vi "Facade.vi"(0 "Data In":T7={"Y"={"Numeric"=25.0, "Numeric"=0.0, "Numeric"=0.0}, "end_timer"=TRUE} {"Y" scale=0.0..500.0 scale format="%#_5g"}, 2 "Display State In":T3={"SP_Source"={"connect"=FALSE, "SP_Source"=enum."initialize", "SP_Set"=0.0, "SP"=0.0}, "Write"=FALSE, "button state"=enum."init", "reset_timer"=FALSE, "load_timer"=FALSE, "end_timer"=TRUE, "Time"=0, "scale maximum"=100.0}, 3 "Container State":T6) -> (6 "Data Out":T7={"Y"={"Numeric"=25.0, "Numeric"=0.0, "Numeric"=0.0}, "end_timer"=TRUE} {"Y" scale=0.0..500.0 scale format="%#_5g"}, 7 "Display State Out":T3={"SP_Source"={"connect"=FALSE, "SP_Source"=enum."initialize", "SP_Set"=0.0, "SP"=0.0}, "Write"=FALSE, "button state"=enum."init", "reset_timer"=FALSE, "load_timer"=FALSE, "end_timer"=TRUE, "Time"=0, "scale maximum"=100.0}, 8 "Action":T2)   [LabVIEW 2019, in "Y.xctl"]
uses:
  Y.xctl
  Data.ctl
  <vilib>/_xctls/Container State.ctl
  State.ctl
  Heating/ctl/Y_source.ctl
  Y_controlState.ctl
  <vilib>/_xctls/Action.ctl
  <vilib>/_xctls/XControlSupport.lvlib
  Timer Delay/Timers.lvlib
  Heating/Heating.lvlib
panel:
  in  "setpoint":T1(slide) caption="oC" scale=0.0..500.0 scale format="%#_5g"
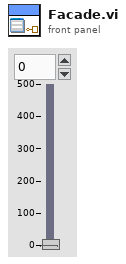
[diagram p1: front panel]
types:
  T1 = cluster{"Numeric":dbl, "Numeric":dbl, "Numeric":dbl}
  T2 = typedef "XControlSupport.lvlib/Action.ctl" = cluster{"Data Changed?":bool, "State Changed?":bool, "Action Name":string}
  T3 = typedef "Y.xctl/State.ctl" = cluster{"SP_Source":cluster{"connect":bool, "SP_Source":T4, "SP_Set":dbl, "SP":dbl}, "Write":bool, "button state":T5, "reset_timer":bool, "load_timer":bool, "end_timer":bool, "Time":u32, "scale maximum":dbl}
  T4 = typedef "Heating.lvlib/Y_source.ctl" = enum8{"initialize", "local disabled", "local hand", "hand", "auto", "dist"}
  T5 = typedef "Y.xctl/Y_controlState.ctl" = enum16{"init", "not connect", "local disabled", "local hand", "hand", "value change", "auto", "dist"}
  T6 = typedef "XControlSupport.lvlib/Container State.ctl" = cluster{"Indicator?":bool, "Run Mode?":bool, " Refnum":refnum<vi>}
  T7 = typedef "Y.xctl/Data.ctl" = cluster{"Y":cluster{"Numeric":dbl, "Numeric":dbl, "Numeric":dbl}, "end_timer":bool}
  T8 = enum8{"Enabled", "Disabled", "Disabled and Grayed Out"}
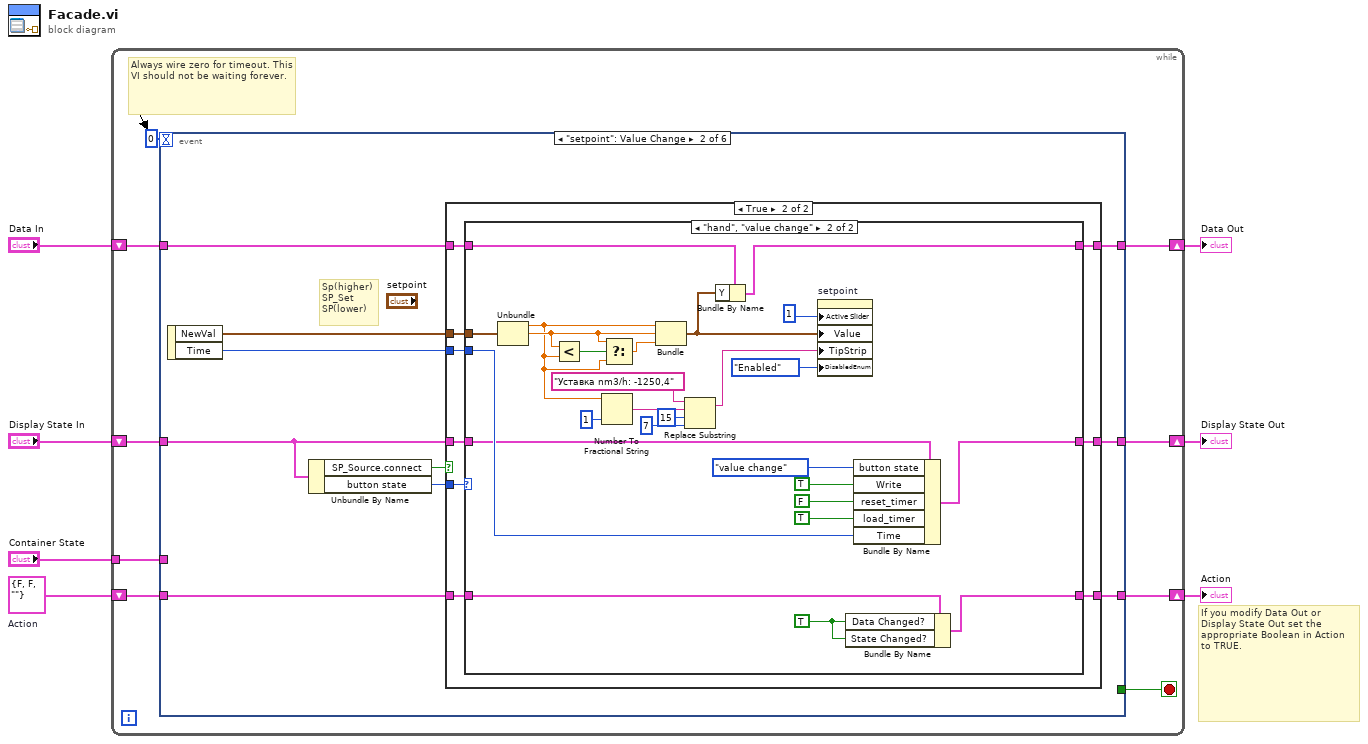
[diagram p0: block diagram]
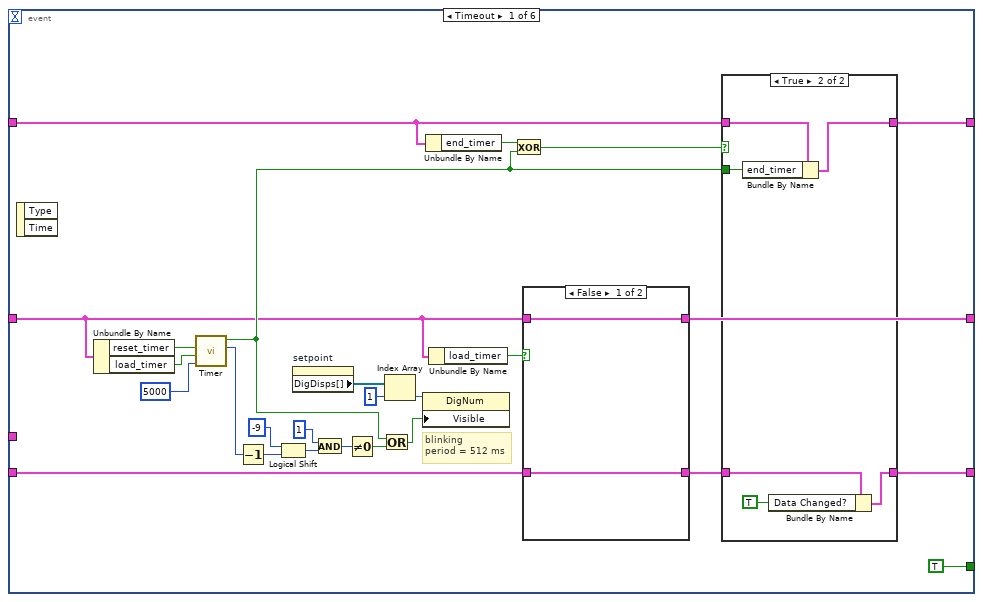
[diagram p2: hidden frame]
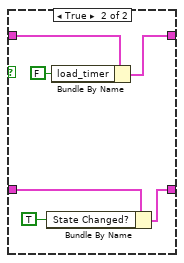
[diagram p4: hidden frame]
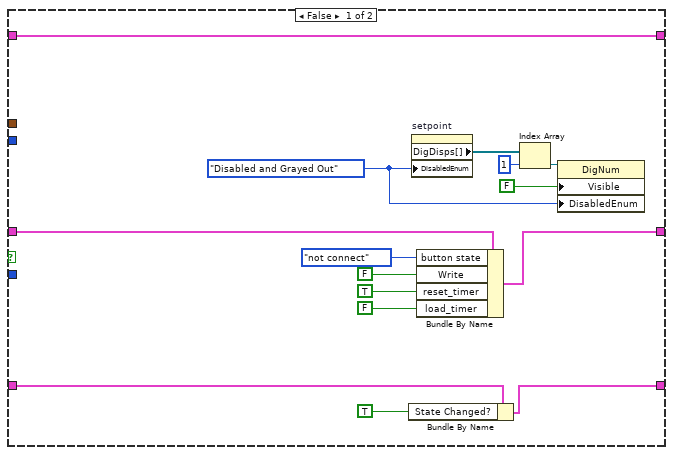
[diagram p5: hidden frame]
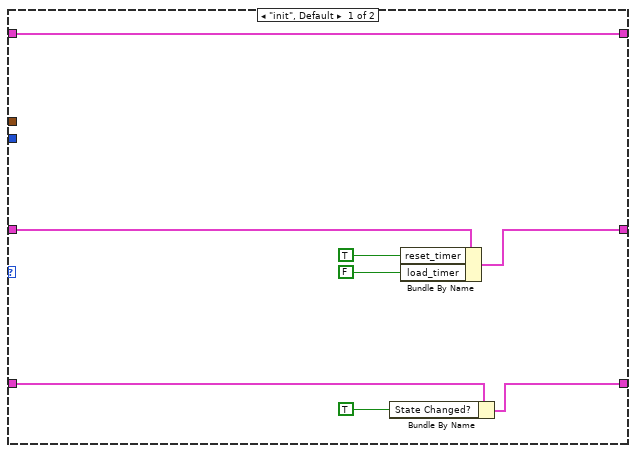
[diagram p6: hidden frame]
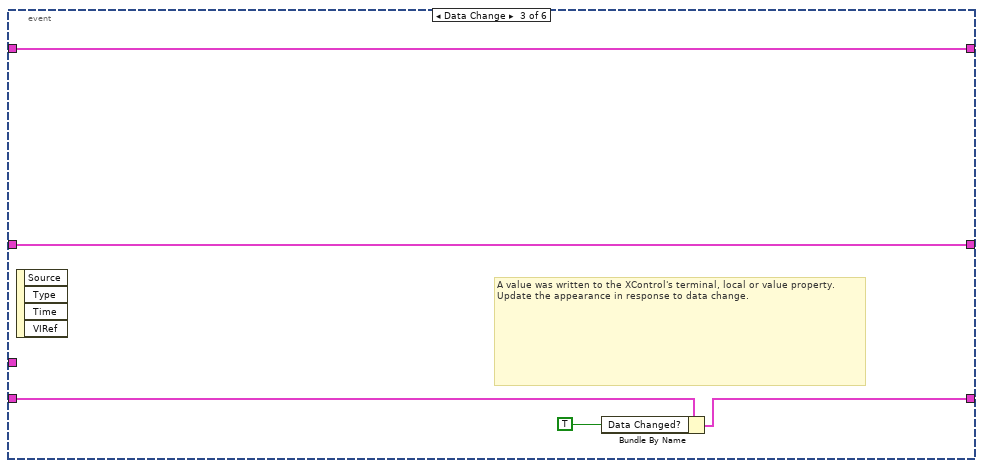
[diagram p7: hidden frame]
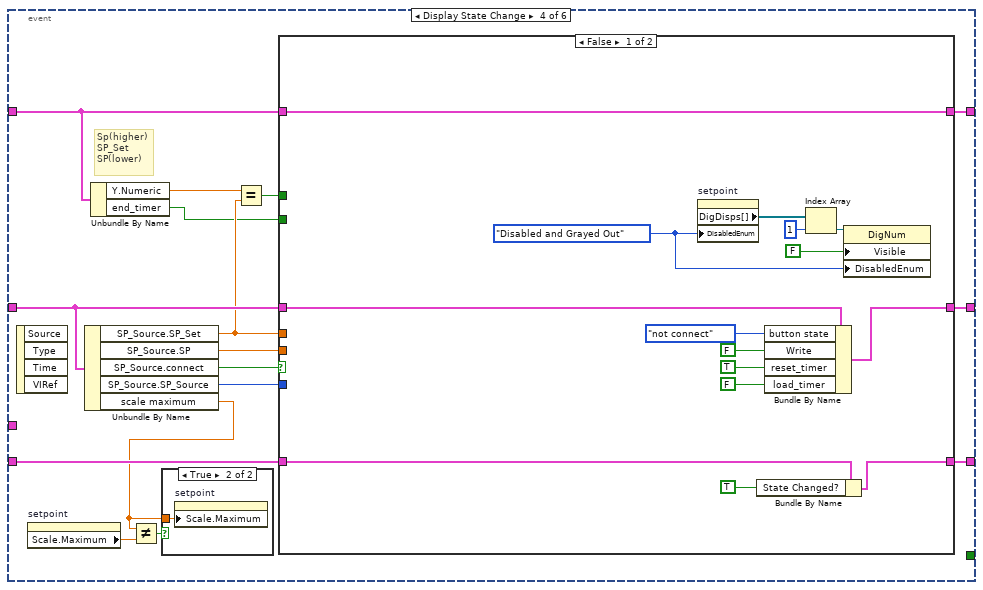
[diagram p8: hidden frame]
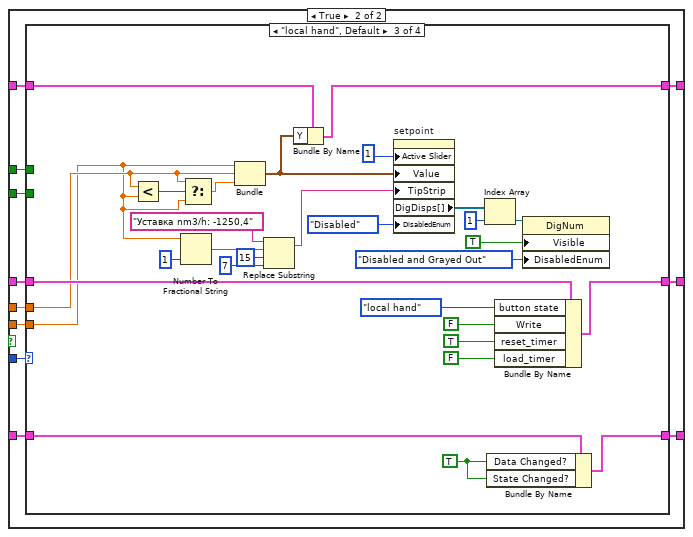
[diagram p10: hidden frame]
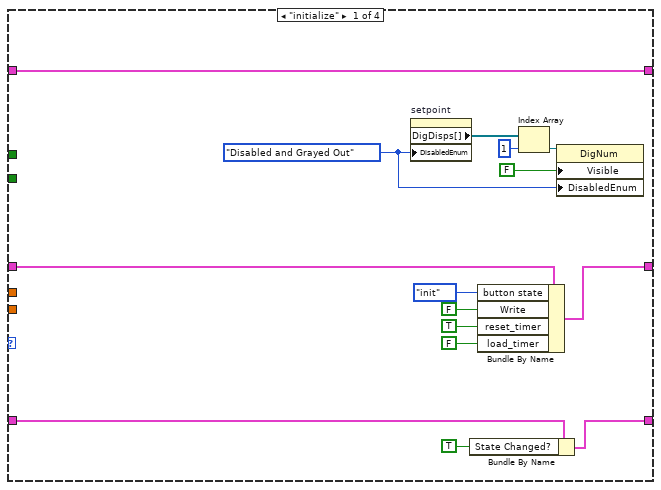
[diagram p11: hidden frame]
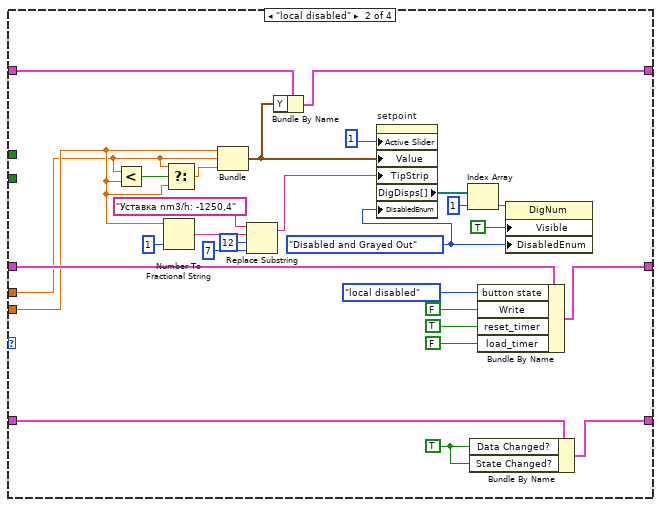
[diagram p12: hidden frame]
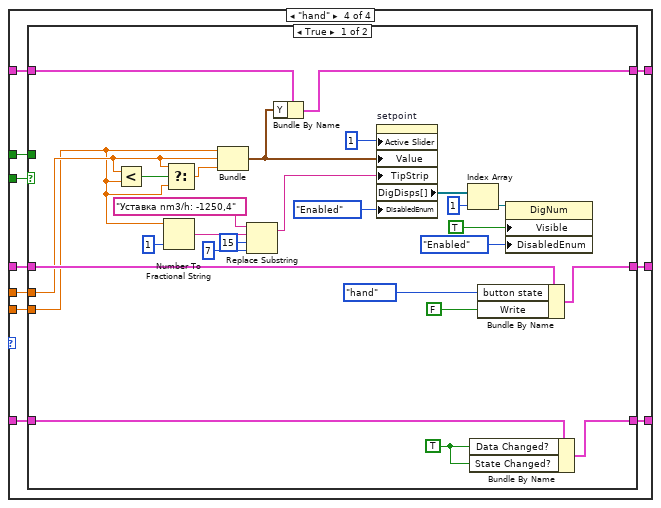
[diagram p13: hidden frame]
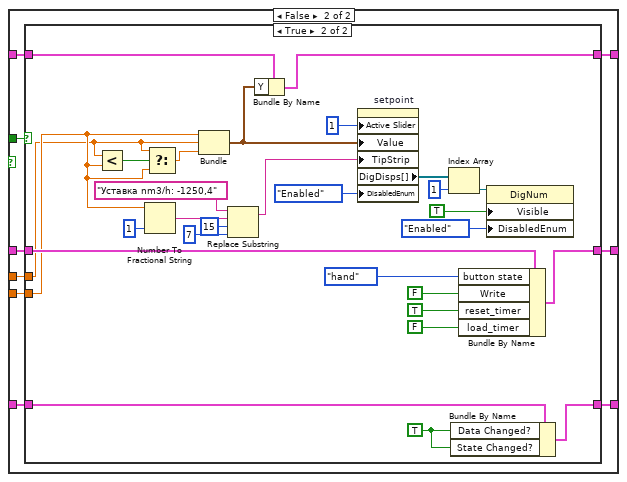
[diagram p14: hidden frame]
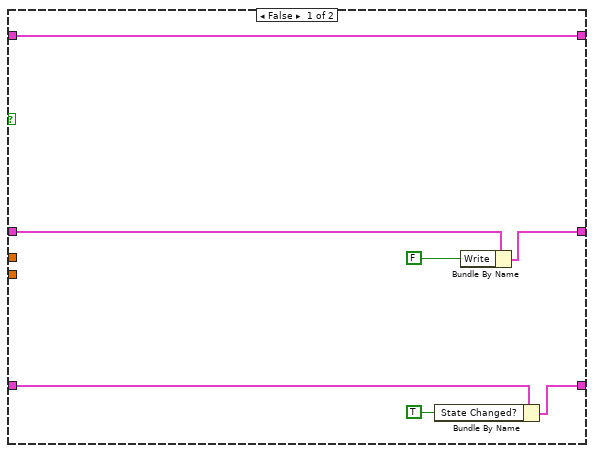
[diagram p15: hidden frame]
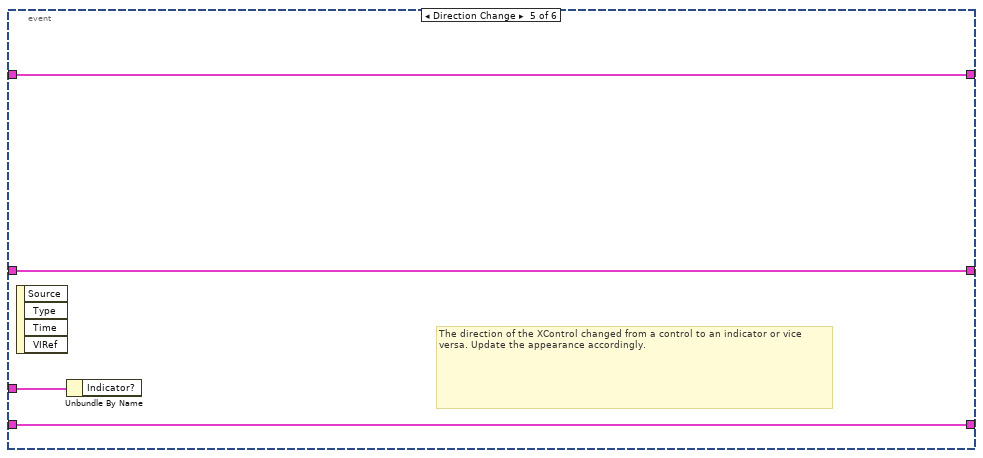
[diagram p16: hidden frame]
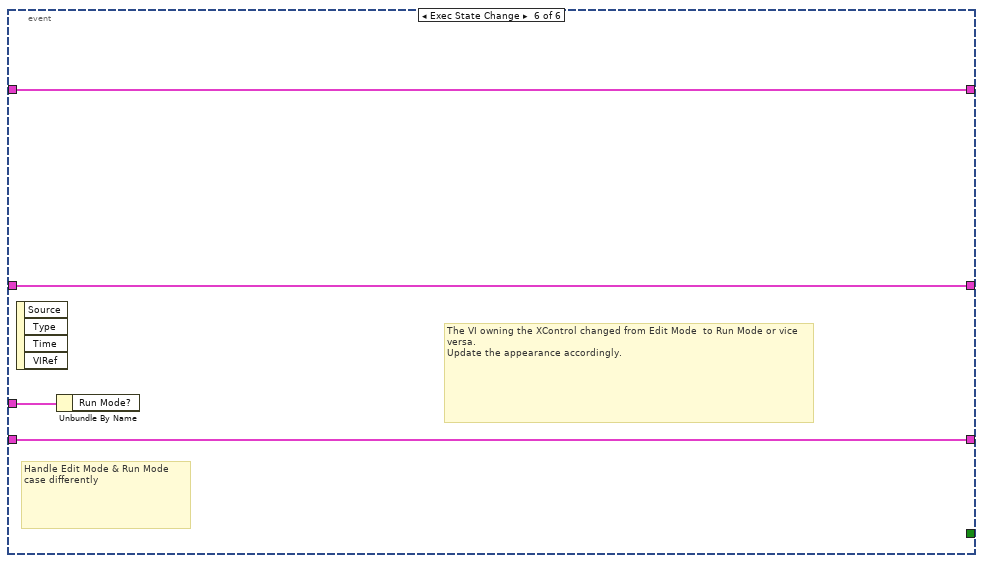
[diagram p17: hidden frame]
diagram:
  w1 = T2 {"Data Changed?"=FALSE, "State Changed?"=FALSE, "Action Name"=""}  # Action
  # "If you modify Data Out or\nDisplay State Out set the\nappropriate Boolean in Action\nto TRUE."
  n1 = while {
    shift-right: [w9] -> w4
    shift-left: "Display State In" -> [w16]
    tunnel: "Container State" -> [w13]
    shift-right: [w8] -> w7
    shift-left: "Data In" -> [w12]
    shift-right: [w10] -> w2
    shift-left: w1 -> [w11]
    stop <- w15 stop-if-true
    # "Always wire zero for timeout. This\nVI should not be waiting forever."
    n2 = event shown="[1] \"setpoint\": Value Change" {
      selector: _ -> [_ _ _ _ _ _]
      dyn-events: _ -> [_ _ _ _ _ _]
      timeout: 0 -> [_ _ _ _ _ _]
      tunnel: w16 -> [w19 w63 w130 w142 w331 w335]
      tunnel: [w25 w68 w130 w146 w331 w335] -> w9
      tunnel: [TRUE _ _ _ _ _] -> w15
      tunnel: w13 -> [_ _ _ _ w332 w336]
      tunnel: w12 -> [w24 w67 w131 w134 w330 w334]
      tunnel: [w17 w66 w131 w147 w330 w334] -> w8
      tunnel: [w21 w64 w128 w144 w329 w333] -> w10
      tunnel: w11 -> [w22 w65 w127 w145 w329 w333]
      event Timeout {
        # "blinking\nperiod = 512 ms"
        n3 = event-data() -> ()  [unwired: 1 in, 2 out]
        n4 = Unbundle By Name(w19) -> ("reset_timer"=w41:bool, "load_timer"=w40:bool)
        n5 = call "Timer.vi"("ms"=5000, "Load (F)"=w40, "Reset (F)"=w41) -> ("t ms"=w39:u32, "End"=w23:bool)  [unwired: 6 in]
        n6 = Decrement(x=w39) -> (x-1=w36:u32)
        n7 = Logical Shift(y=i16 -9, x=w36) -> (x << y=w34:u32)
        n8 = property on="setpoint" class="Slide (strict)"() -> ("DigDisps[]"=w28:refnum<vi>[])  [unwired: 2 in, 2 out]
        n9 = And(x=u32 1 ("y"), y=w34) -> (x .and. y?=w32:u32)
        n10 = Not Equal To 0?(x=w32) -> (x != 0?=w37:bool)
        n11 = Or(x=w23, y=w37) -> (x .or. y?=w29:bool)
        n12 = Index Array(array=w28, index=1) -> (element=w31:refnum<vi>)
        n13 = property class="DigNum"(reference=w31, "Visible"=w29) -> ()  [unwired: 1 in, 2 out]
        n14 = Unbundle By Name(w24) -> ("end_timer"=w18:bool)
        n15 = Unbundle By Name(w19) -> ("load_timer"=w20:bool)
        n16 = Exclusive Or(1:w23, 2:w18) -> (0:w27:bool)
        n17 = case shown="False" w20 {
          tunnel: [w52 w58] -> w25
          tunnel: w19 -> [w52 w56]
          tunnel: w22 -> [w51 w54]
          tunnel: [w51 w53] -> w26
          frame False {
          }
          frame True {
            n18 = Bundle By Name(cluster=w54, "State Changed?"=TRUE ("Data Changed?")) -> (w53:T2)
            n19 = Bundle By Name(cluster=w56, "load_timer"=FALSE) -> (w58:T3)
          }
        }
        n20 = case shown="True" w27 {
          tunnel: [w43 w50] -> w17
          tunnel: w24 -> [w43 w49]
          tunnel: w23 -> [_ w48]
          tunnel: w26 -> [w44 w46]
          tunnel: [w44 w45] -> w21
          frame False {
          }
          frame True {
            n21 = Bundle By Name(cluster=w49, "end_timer"=w48) -> (w50:T7)
            n22 = Bundle By Name(cluster=w46, "Data Changed?"=TRUE) -> (w45:T2)
          }
        }
      }
      event "setpoint": Value Change {
        # "Sp(higher)\nSP_Set\nSP(lower)"
        n23 = event-data() -> ("NewVal"=w60:T1, "Time"=w59:u32)  [unwired: 1 in]
        n24 = Unbundle By Name(w63) -> ("SP_Source.connect"=w62:bool, "button state"=w61:T5)
        n25 = case shown="True" w62 {
          tunnel: w61 -> [_ w92]
          tunnel: w63 -> [w82 w91]
          tunnel: [w81 w90] -> w68
          tunnel: w67 -> [w74 w89]
          tunnel: [w74 w88] -> w66
          tunnel: w65 -> [w79 w86]
          tunnel: [w78 w87] -> w64
          tunnel: w60 -> [_ w85]
          tunnel: w59 -> [_ w84]
          frame False {
            w70 = T8."Disabled and Grayed Out" ("Disabled")
            n26 = Bundle By Name(cluster=w79, "State Changed?"=TRUE ("Data Changed?")) -> (w78:T2)
            n27 = property on="setpoint" class="Slide (strict)"("DisabledEnum"=w70) -> ("DigDisps[]"=w69:refnum<vi>[])  [unwired: 2 in, 2 out]
            n28 = Bundle By Name(cluster=w82, "button state"=Y_controlState."not connect" ("f 3"), "Write"=FALSE ("Z_ASwitch"), "reset_timer"=TRUE ("Z_ASwitch"), "load_timer"=FALSE ("Z_ASwitch")) -> (w81:T3)
            n29 = Index Array(array=w69, index=1) -> (element=w73:refnum<vi>)
            n30 = property class="DigNum"(reference=w73, "Visible"=FALSE ("Z_ASwitch"), "DisabledEnum"=w70) -> ()  [unwired: 1 in, 2 out]
          }
          frame True {
            n31 = case shown="\"hand\", \"value change\"" w92 {
              tunnel: w91 -> [w99 w104]
              tunnel: [w98 w126] -> w90
              tunnel: w89 -> [w93 w103]
              tunnel: [w93 w101] -> w88
              tunnel: [w95 w124] -> w87
              tunnel: w86 -> [w96 w125]
              tunnel: w85 -> [_ w109]
              tunnel: w84 -> [_ w105]
              frame "init", Default {
                # "local hand"
                n32 = Bundle By Name(cluster=w96, "State Changed?"=TRUE ("Data Changed?")) -> (w95:T2)
                n33 = Bundle By Name(cluster=w99, "reset_timer"=TRUE, "load_timer"=FALSE) -> (w98:T3)
              }
              frame "hand", "value change" {
                w120 = TRUE ("Data Changed?")
                # "local hand"
                n34 = Unbundle(w109) -> ("Numeric"=w107:dbl, "Numeric"=w108:dbl)  [unwired: 1 out]
                n35 = Less?(x=w108, y=w107) -> (x < y?=w112:bool)
                n36 = Number To Fractional String(number=w107, precision (6)=i16 1) -> (F-format string=w115:string)  [unwired: 2 in]
                n37 = Select(t=w108, s=w112, f=w107) -> (s? t:f=w111:dbl)
                n38 = Bundle("Numeric"=w107, "Numeric"=w108, "Numeric"=w111) -> (w102:T1)  [unwired: 1 in]
                n39 = Replace Substring(2:7 ("length (len. of substring)"), 3:15 ("offset (0)"), 4:w115, 5:"Уставка nm3/h: -1250,4") -> (1:w106:string)  [unwired: 1 out]
                n40 = Bundle By Name(cluster=w103, "Y"=w102) -> (w101:T7)
                n41 = property on="setpoint" class="Slide (strict)"("Active Slider"=1, "Value"=w102, "TipStrip"=w106, "DisabledEnum"=T8."Enabled" ("Disabled")) -> ()  [unwired: 2 in, 2 out]
                n42 = Bundle By Name(cluster=w125, "Data Changed?"=w120, "State Changed?"=w120) -> (w124:T2)
                n43 = Bundle By Name(cluster=w104, "button state"=Y_controlState."value change" ("f 3"), "Write"=TRUE ("Z_ASwitch"), "reset_timer"=FALSE ("Z_ASwitch"), "load_timer"=TRUE ("Z_ASwitch"), "Time"=w105) -> (w126:T3)
              }
            }
          }
        }
      }
      event Data Change {
        # "A value was written to the XControl's terminal, local or value property.\nUpdate the appearance in response to data change."
        n44 = event-data() -> ()  [unwired: 1 in, 4 out]
        n45 = Bundle By Name(cluster=w127, "Data Changed?"=TRUE) -> (w128:T2)
      }
      event Display State Change {
        # "Sp(higher)\nSP_Set\nSP(lower)"
        n46 = event-data() -> ()  [unwired: 1 in, 4 out]
        n47 = property on="setpoint" class="Slide (strict)"() -> ("Scale.Maximum"=w137:dbl)  [unwired: 2 in, 2 out]
        n48 = Unbundle By Name(w142) -> ("SP_Source.SP_Set"=w138:dbl, "SP_Source.SP"=w139:dbl, "SP_Source.connect"=w143:bool, "SP_Source.SP_Source"=w141:T4, "scale maximum"=w136:dbl)
        n49 = Unbundle By Name(w134) -> ("Y.Numeric"=w133:dbl, "end_timer"=w132:bool)
        n50 = Not Equal?(x=w136, y=w137) -> (x != y?=w135:bool)
        n51 = case shown="True" w135 {
          tunnel: w136 -> [_ w148]
          frame False {
          }
          frame True {
            n52 = property on="setpoint" class="Slide (strict)"("Scale.Maximum"=w148) -> ()  [unwired: 2 in, 2 out]
          }
        }
        n53 = Equal?(x=w133, y=w138) -> (x = y?=w140:bool)
        n54 = case shown="False" w143 {
          tunnel: w141 -> [_ w174]
          tunnel: w142 -> [w162 w173]
          tunnel: [w161 w172] -> w146
          tunnel: w134 -> [w150 w171]
          tunnel: [w150 w170] -> w147
          tunnel: w145 -> [w159 w168]
          tunnel: [w158 w169] -> w144
          tunnel: w132 -> [_ w167]
          tunnel: w139 -> [_ w166]
          tunnel: w140 -> [_ w165]
          tunnel: w138 -> [_ w164]
          frame False {
            w149 = T8."Disabled and Grayed Out" ("Disabled")
            n55 = property on="setpoint" class="Slide (strict)"("DisabledEnum"=w149) -> ("DigDisps[]"=w153:refnum<vi>[])  [unwired: 2 in, 2 out]
            n56 = Bundle By Name(cluster=w159, "State Changed?"=TRUE ("Data Changed?")) -> (w158:T2)
            n57 = Bundle By Name(cluster=w162, "button state"=Y_controlState."not connect" ("f 3"), "Write"=FALSE ("Z_ASwitch"), "reset_timer"=TRUE ("Z_ASwitch"), "load_timer"=FALSE ("Z_ASwitch")) -> (w161:T3)
            n58 = Index Array(array=w153, index=1) -> (element=w154:refnum<vi>)
            n59 = property class="DigNum"(reference=w154, "Visible"=FALSE ("Z_ASwitch"), "DisabledEnum"=w149) -> ()  [unwired: 1 in, 2 out]
          }
          frame True {
            n60 = case shown="\"local hand\", Default" w174 {
              tunnel: w173 -> [w189 w217 w246 w256]
              tunnel: [w188 w216 w245 w255] -> w172
              tunnel: w171 -> [w175 w192 w220 w249]
              tunnel: [w175 w190 w218 w250] -> w170
              tunnel: [w186 w214 w243 w253] -> w169
              tunnel: w168 -> [w187 w215 w244 w254]
              tunnel: w167 -> [_ _ _ w252]
              tunnel: w166 -> [_ w195 w222 w251]
              tunnel: w165 -> [_ _ _ w248]
              tunnel: w164 -> [_ w194 w223 w247]
              frame "initialize" {
                w180 = T8."Disabled and Grayed Out" ("Disabled")
                # "local hand"
                n61 = property on="setpoint" class="Slide (strict)"("DisabledEnum"=w180) -> ("DigDisps[]"=w178:refnum<vi>[])  [unwired: 2 in, 2 out]
                n62 = Bundle By Name(cluster=w187, "State Changed?"=TRUE ("Data Changed?")) -> (w186:T2)
                n63 = Bundle By Name(cluster=w189, "button state"=Y_controlState."init" ("f 3"), "Write"=FALSE ("Z_ASwitch"), "reset_timer"=TRUE ("Z_ASwitch"), "load_timer"=FALSE ("Z_ASwitch")) -> (w188:T3)
                n64 = Index Array(array=w178, index=1) -> (element=w179:refnum<vi>)
                n65 = property class="DigNum"(reference=w179, "Visible"=FALSE ("Z_ASwitch"), "DisabledEnum"=w180) -> ()  [unwired: 1 in, 2 out]
              }
              frame "local disabled" {
                w193 = T8."Disabled and Grayed Out" ("Disabled")
                w209 = TRUE ("Data Changed?")
                # "local hand"
                n66 = Less?(x=w194, y=w195) -> (x < y?=w200:bool)
                n67 = Number To Fractional String(number=w195, precision (6)=i16 1) -> (F-format string=w203:string)  [unwired: 2 in]
                n68 = Select(t=w194, s=w200, f=w195) -> (s? t:f=w199:dbl)
                n69 = Bundle("SP"=w195, "SP_Set"=w194, "SP"=w199) -> (w191:cluster{"SP":dbl, "SP_Set":dbl, "SP":dbl})  [unwired: 1 in]
                n70 = Replace Substring(2:7 ("length (len. of substring)"), 3:12 ("offset (0)"), 4:w203, 5:"Уставка nm3/h: -1250,4") -> (1:w198:string)  [unwired: 1 out]
                n71 = Bundle By Name(cluster=w192, "Y"=w191) -> (w190:T7)
                n72 = property on="setpoint" class="Slide (strict)"("Active Slider"=1, "Value"=w191, "TipStrip"=w198, "DisabledEnum"=w193) -> ("DigDisps[]"=w196:refnum<vi>[])  [unwired: 2 in, 2 out]
                n73 = Index Array(array=w196, index=1) -> (element=w208:refnum<vi>)
                n74 = Bundle By Name(cluster=w215, "Data Changed?"=w209, "State Changed?"=w209) -> (w214:T2)
                n75 = Bundle By Name(cluster=w217, "button state"=Y_controlState."local disabled" ("f 3"), "Write"=FALSE ("Z_ASwitch"), "reset_timer"=TRUE ("Z_ASwitch"), "load_timer"=FALSE ("Z_ASwitch")) -> (w216:T3)
                n76 = property class="DigNum"(reference=w208, "Visible"=TRUE ("Z_ASwitch"), "DisabledEnum"=w193) -> ()  [unwired: 1 in, 2 out]
              }
              frame "local hand", Default {
                w238 = TRUE ("Data Changed?")
                # "local hand"
                n77 = Less?(x=w223, y=w222) -> (x < y?=w227:bool)
                n78 = Number To Fractional String(number=w222, precision (6)=i16 1) -> (F-format string=w230:string)  [unwired: 2 in]
                n79 = Select(t=w223, s=w227, f=w222) -> (s? t:f=w226:dbl)
                n80 = Bundle("SP"=w222, "SP_Set"=w223, "SP"=w226) -> (w219:cluster{"SP":dbl, "SP_Set":dbl, "SP":dbl})  [unwired: 1 in]
                n81 = Replace Substring(2:7 ("length (len. of substring)"), 3:15 ("offset (0)"), 4:w230, 5:"Уставка nm3/h: -1250,4") -> (1:w221:string)  [unwired: 1 out]
                n82 = Bundle By Name(cluster=w220, "Y"=w219) -> (w218:T7)
                n83 = property on="setpoint" class="Slide (strict)"("Active Slider"=1, "Value"=w219, "TipStrip"=w221, "DisabledEnum"=T8."Disabled" ("Disabled")) -> ("DigDisps[]"=w224:refnum<vi>[])  [unwired: 2 in, 2 out]
                n84 = Index Array(array=w224, index=1) -> (element=w237:refnum<vi>)
                n85 = Bundle By Name(cluster=w244, "Data Changed?"=w238, "State Changed?"=w238) -> (w243:T2)
                n86 = Bundle By Name(cluster=w246, "button state"=Y_controlState."local hand" ("f 3"), "Write"=FALSE ("Z_ASwitch"), "reset_timer"=TRUE ("Z_ASwitch"), "load_timer"=FALSE ("Z_ASwitch")) -> (w245:T3)
                n87 = property class="DigNum"(reference=w237, "Visible"=TRUE ("Z_ASwitch"), "DisabledEnum"=T8."Disabled and Grayed Out" ("Disabled")) -> ()  [unwired: 1 in, 2 out]
              }
              frame "hand" {
                # "local hand"
                n88 = case shown="True" w252 {
                  tunnel: w256 -> [w283 w292]
                  tunnel: [w282 w291] -> w255
                  tunnel: w254 -> [w281 w290]
                  tunnel: [w280 w289] -> w253
                  tunnel: w251 -> [w261 w286]
                  tunnel: [w259 w288] -> w250
                  tunnel: w249 -> [w258 w287]
                  tunnel: w248 -> [_ w285]
                  tunnel: w247 -> [w262 w284]
                  frame True {
                    w277 = TRUE ("Data Changed?")
                    n89 = Less?(x=w262, y=w261) -> (x < y?=w265:bool)
                    n90 = Number To Fractional String(number=w261, precision (6)=i16 1) -> (F-format string=w268:string)  [unwired: 2 in]
                    n91 = Select(t=w262, s=w265, f=w261) -> (s? t:f=w264:dbl)
                    n92 = Bundle("SP"=w261, "SP_Set"=w262, "SP"=w264) -> (w257:cluster{"SP":dbl, "SP_Set":dbl, "SP":dbl})  [unwired: 1 in]
                    n93 = Replace Substring(2:7 ("length (len. of substring)"), 3:15 ("offset (0)"), 4:w268, 5:"Уставка nm3/h: -1250,4") -> (1:w260:string)  [unwired: 1 out]
                    n94 = Bundle By Name(cluster=w258, "Y"=w257) -> (w259:T7)
                    n95 = property on="setpoint" class="Slide (strict)"("Active Slider"=1, "Value"=w257, "TipStrip"=w260, "DisabledEnum"=T8."Enabled" ("Disabled")) -> ("DigDisps[]"=w274:refnum<vi>[])  [unwired: 2 in, 2 out]
                    n96 = Index Array(array=w274, index=1) -> (element=w275:refnum<vi>)
                    n97 = Bundle By Name(cluster=w281, "Data Changed?"=w277, "State Changed?"=w277) -> (w280:T2)
                    n98 = Bundle By Name(cluster=w283, "button state"=Y_controlState."hand" ("f 3"), "Write"=FALSE ("Z_ASwitch")) -> (w282:T3)
                    n99 = property class="DigNum"(reference=w275, "Visible"=TRUE ("Z_ASwitch"), "DisabledEnum"=T8."Enabled" ("Disabled")) -> ()  [unwired: 1 in, 2 out]
                  }
                  frame False {
                    n100 = case shown="True" w285 {
                      tunnel: w292 -> [w295 w328]
                      tunnel: [w294 w327] -> w291
                      tunnel: w290 -> [w298 w326]
                      tunnel: [w296 w325] -> w289
                      tunnel: [w299 w301] -> w288
                      tunnel: w287 -> [w299 w302]
                      tunnel: w286 -> [_ w306]
                      tunnel: w284 -> [_ w305]
                      frame False {
                        n101 = Bundle By Name(cluster=w298, "State Changed?"=TRUE ("Data Changed?")) -> (w296:T2)
                        n102 = Bundle By Name(cluster=w295, "Write"=FALSE ("Z_ASwitch")) -> (w294:T3)
                      }
                      frame True {
                        w322 = TRUE ("Data Changed?")
                        n103 = Less?(x=w305, y=w306) -> (x < y?=w308:bool)
                        n104 = Number To Fractional String(number=w306, precision (6)=i16 1) -> (F-format string=w311:string)  [unwired: 2 in]
                        n105 = Select(t=w305, s=w308, f=w306) -> (s? t:f=w307:dbl)
                        n106 = Bundle("SP"=w306, "SP_Set"=w305, "SP"=w307) -> (w300:cluster{"SP":dbl, "SP_Set":dbl, "SP":dbl})  [unwired: 1 in]
                        n107 = Replace Substring(2:7 ("length (len. of substring)"), 3:15 ("offset (0)"), 4:w311, 5:"Уставка nm3/h: -1250,4") -> (1:w303:string)  [unwired: 1 out]
                        n108 = Bundle By Name(cluster=w302, "Y"=w300) -> (w301:T7)
                        n109 = property on="setpoint" class="Slide (strict)"("Active Slider"=1, "Value"=w300, "TipStrip"=w303, "DisabledEnum"=T8."Enabled" ("Disabled")) -> ("DigDisps[]"=w319:refnum<vi>[])  [unwired: 2 in, 2 out]
                        n110 = Index Array(array=w319, index=1) -> (element=w320:refnum<vi>)
                        n111 = Bundle By Name(cluster=w326, "Data Changed?"=w322, "State Changed?"=w322) -> (w325:T2)
                        n112 = Bundle By Name(cluster=w328, "button state"=Y_controlState."hand" ("f 3"), "Write"=FALSE ("Z_ASwitch"), "reset_timer"=TRUE ("Z_ASwitch"), "load_timer"=FALSE ("Z_ASwitch")) -> (w327:T3)
                        n113 = property class="DigNum"(reference=w320, "Visible"=TRUE ("Z_ASwitch"), "DisabledEnum"=T8."Enabled" ("Disabled")) -> ()  [unwired: 1 in, 2 out]
                      }
                    }
                  }
                }
              }
            }
          }
        }
      }
      event Direction Change {
        # "The direction of the XControl changed from a control to an indicator or vice versa. Update the appearance accordingly."
        n114 = event-data() -> ()  [unwired: 1 in, 4 out]
        n115 = Unbundle By Name(w332) -> ()  [unwired: 1 out]
      }
      event Exec State Change {
        # "The VI owning the XControl changed from Edit Mode  to Run Mode or vice versa.\nUpdate the appearance accordingly."
        # "Handle Edit Mode & Run Mode\ncase differently"
        n116 = event-data() -> ()  [unwired: 1 in, 4 out]
        n117 = Unbundle By Name(w336) -> ()  [unwired: 1 out]
      }
    }
  }
  "Display State Out" <- w4
  "Data Out" <- w7
  "Action" <- w2
